vi "VectorField1009.vi"   [LabVIEW 2013]
uses:
  <vilib>/Heliosphere Research LLC/Advanced Plotting Toolkit/api_plotting/VectorFieldProperties.ctl
  <vilib>/Heliosphere Research LLC/Advanced Plotting Toolkit/typedefs/PlotColor.ctl
  <vilib>/Heliosphere Research LLC/Advanced Plotting Toolkit/properties/Colormap.ctl
  <vilib>/Heliosphere Research LLC/Advanced Plotting Toolkit/properties/Colormap_Map.ctl
  <vilib>/Heliosphere Research LLC/Advanced Plotting Toolkit/properties/Colormap_Scaling.ctl
  <vilib>/Heliosphere Research LLC/Advanced Plotting Toolkit/properties/Display.ctl
  <vilib>/Heliosphere Research LLC/Advanced Plotting Toolkit/Advanced Plotting Toolkit.lvlib
types:
  T1 = typedef "Advanced Plotting Toolkit.lvlib/VectorFieldProperties.ctl" = cluster{"Color":T2, "Arrow Scale":dbl, "Colormap":T3, "Display":T6}
  T2 = typedef "Advanced Plotting Toolkit.lvlib/PlotColor.ctl" = u32
  T3 = typedef "Advanced Plotting Toolkit.lvlib/Colormap.ctl" = cluster{"Map":T4, "Value Min":dbl, "Value Max":dbl, "Scaling":T5, "Reverse":bool}
  T4 = typedef "Advanced Plotting Toolkit.lvlib/Colormap_Map.ctl" = enum16{"Automatic", "Rainbow", "Hot and Cold", "White-Black", "White-Blue", "White-Green", "White-Red", "Fire", "Water", "Earth", "Air", "Pastel", "Banded", "Stepped"}
  T5 = typedef "Advanced Plotting Toolkit.lvlib/Colormap_Scaling.ctl" = enum16{"Default"}
  T6 = typedef "Advanced Plotting Toolkit.lvlib/Display.ctl" = cluster{"Alpha":dbl, "Z Order":dbl}
  T7 = typedef "Advanced Plotting Toolkit.lvlib/PlotID.ctl" = i32
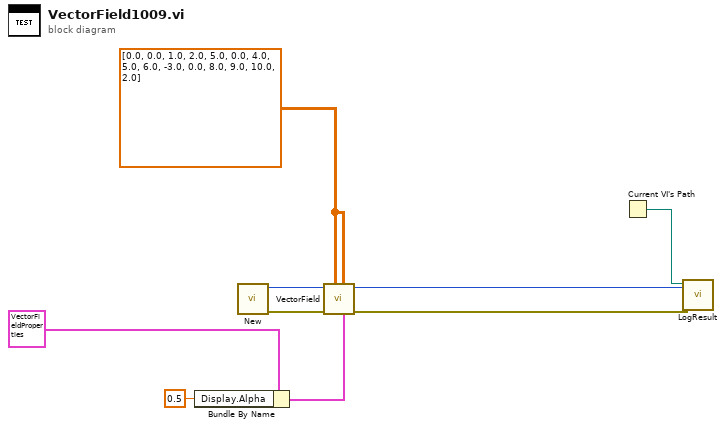
[diagram p0: block diagram]
diagram:
  w8 = dbl[][] [[0.0, 0.0, 1.0, 2.0, 5.0], [0.0, 4.0, 5.0, 6.0, -3.0], [0.0, 8.0, 9.0, 10.0, 2.0]] ("Data")
  n1 = Bundle By Name(cluster=T1 {"Color"=2147483647, "Arrow Scale"=nan, "Colormap"={"Map"=enum."Automatic", "Value Min"=nan, "Value Max"=nan, "Scaling"=enum."Default", "Reverse"=FALSE}, "Display"={"Alpha"=nan, "Z Order"=nan}} ("Vector Field Properties"), "Display.Alpha"=0.5) -> (w2:T1)
  n2 = call <vilib>:"New.vi"() -> ("error out"=w6:errorcluster, "Plot ID"=w7:T7)  [unwired: 10 in]
  n3 = call <vilib>:"VectorField.vi"("Properties"=w2, "Y Vector Component"=w8, "X Vector Component"=w8, "error in (no error)"=w6, "Plot ID"=w7) -> ("error out"=w4:errorcluster, "Plot ID Out"=w5:T7)  [unwired: 5 in]
  n4 = Current VI's Path() -> (path=w9:path)
  n5 = call "LogResult.vi"("Test Result"=w4, "Test Artifact"=w5, "VI Path"=w9) -> ()  [unwired: 9 in]
